vi "Read TDATA Core.vi"(11 "niInstr AXI4-Stream Reader FXP64x2 v1 FPGA in":refnum<class "niInstr AXI4-Stream Reader FXP64x2 v1 FPGA.lvclass">) -> (2 "tdata value":bool[](array[boolean]), 3 "niInstr AXI4-Stream Reader FXP64x2 v1 FPGA out":refnum<class "niInstr AXI4-Stream Reader FXP64x2 v1 FPGA.lvclass">)   [LabVIEW 2015, in "niInstr AXI4-Stream Reader FXP64x2 v1 FPGA.lvclass"]
doc: "<B>Input Parameters</B>\n\n<B>niInstr AXI4-Stream Reader FXP64x2 v1 FPGA in</B> takes in a reference to the AXI4-Stream Reader from the previous VI.\n\n<B>Output Parameters</B>\n\n<B>tdata value</B> is the value in the returned TDATA."
uses:
  <instrlib>/_niInstr/CLIP Adapters/v1/FPGA/AXI4-Stream/Reader FXP64x2/niInstr AXI4-Stream Reader FXP64x2 v1 FPGA.lvclass
  <instrlib>/_niInstr/CLIP Adapters/v1/FPGA/AXI4-Stream/Reader FXP64x2/niInstr AXI4-Stream Reader FXP64x2 v1 FPGA.lvclass/niInstr AXI4-Stream Reader FXP64x2 v1 FPGA.ctl
  <instrlib>/_niInstr/Data Formatting/v1/FPGA/Private/Convert/U64 array to Boolean Array.vi
  <vilib>/rvi/eio/common/nirviEmuTemplateMethod_errors.vi
  <vilib>/eio/EIONode/EIONode.xnode
  <instrlib>/_niInstr/Data Formatting/v1/FPGA/niInstr Data Formatting v1 FPGA.lvlib
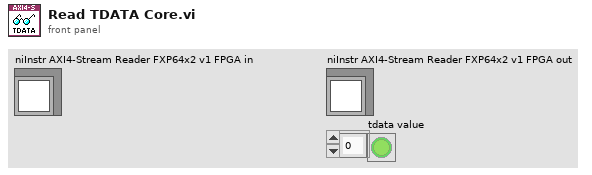
[diagram p1: front panel]
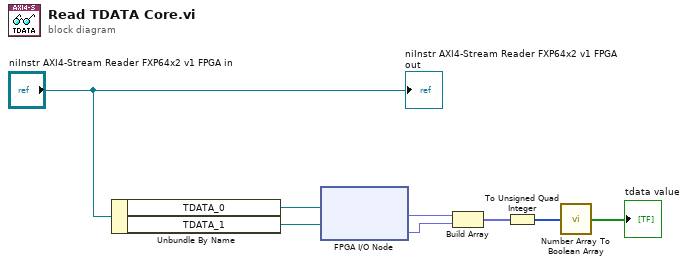
[diagram p0: block diagram]
diagram:
  n1 = Unbundle By Name("niInstr AXI4-Stream Reader FXP64x2 v1 FPGA in") -> ("TDATA_0"=w7:refnum<k21>, "TDATA_1"=w6:refnum<k21>)
  n2 = xnode "FPGA I/O Node"("FPGA I/O In"=w7, "FPGA I/O In"=w6) -> ("I/O Item"=w4:fxp<+,64,64>, "I/O Item"=w3:fxp<+,64,64>)  [unwired: 2 out]
  n3 = Build Array(w4, w3) -> (w2:fxp<+,64,64>[])
  n4 = To Unsigned Quad Integer(1:w2) -> (0:w5:u64[])
  n5 = call-poly <instrlib>:"Number Array To Boolean Array.vi"("data in"=w5) -> ("data out"=→"tdata value":bool[])  [unwired: 14 in]
  "niInstr AXI4-Stream Reader FXP64x2 v1 FPGA out" <- "niInstr AXI4-Stream Reader FXP64x2 v1 FPGA in"
